vi "ATM_displayer.vi"(7 "Message":T1(ring), 9 "Amount":string, 10 "Users Info":string[](array[string])) -> (0 "Right Menu":cluster{string, string, string}, 1 "Left Menu":cluster{string, string, string}, 2 "Message display":string)   [LabVIEW 2025]
doc: "This VI handles the display of the ATM, the Left and Right Menu. It uses two inputs :\nMessage (required) : an Enum of 10 possible values\nUsers Info (optional) : a 1D Array of four strings constant"
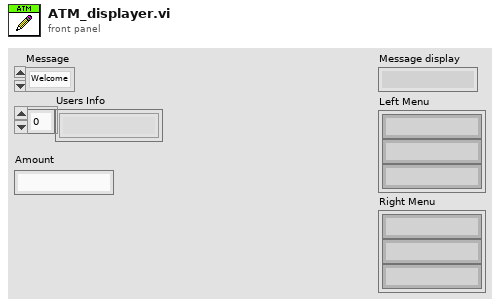
[diagram p1: front panel]
types:
  T1 = enum16{"Welcome", "Main Menu", "Account Verif Failed", "Session Terminate", "Deposit", "Deposit complete", "Withdrawal", "Withdrawal complete", "Withdrawal failed", "Balance Inquiry"}
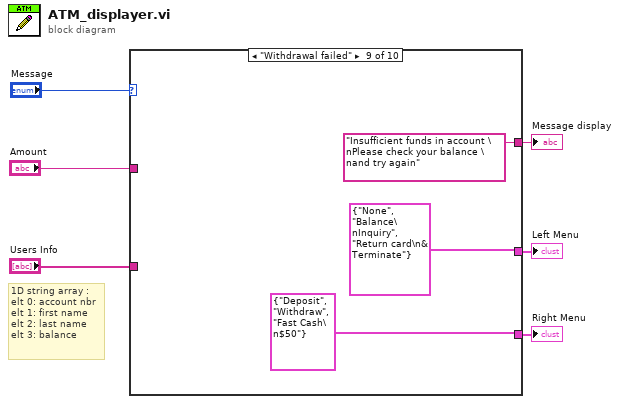
[diagram p0: block diagram]
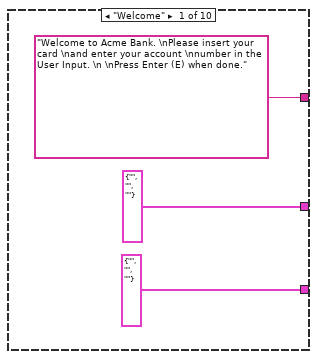
[diagram p2: hidden frame]
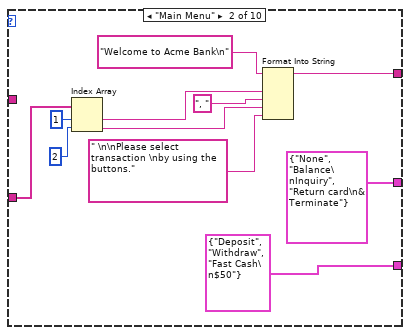
[diagram p3: hidden frame]
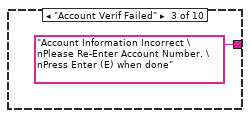
[diagram p4: hidden frame]
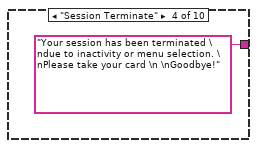
[diagram p5: hidden frame]
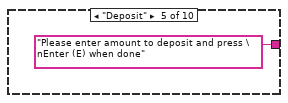
[diagram p6: hidden frame]
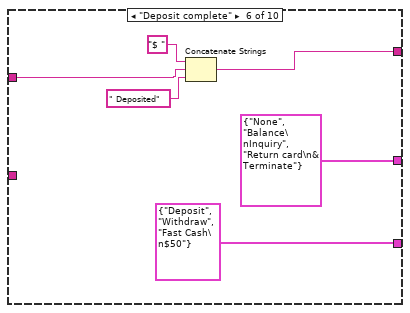
[diagram p7: hidden frame]
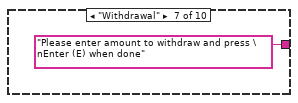
[diagram p8: hidden frame]
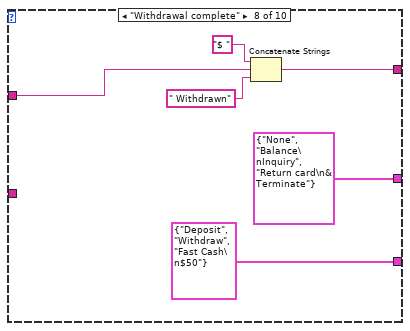
[diagram p9: hidden frame]
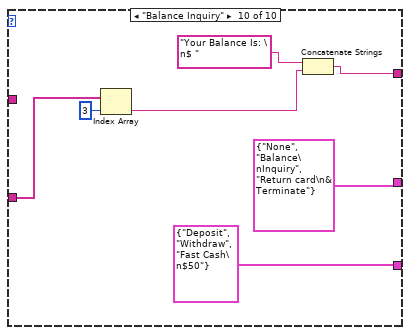
[diagram p10: hidden frame]
diagram:
  # "1D string array :\nelt 0: account nbr\nelt 1: first name\nelt 2: last name\nelt 3: balance"
  n1 = case shown="\"Withdrawal failed\"" "Message" {
    tunnel: ["Welcome to Acme Bank. \nPlease insert your card \nand enter your account \nnumber in the User Input. \n \nPress Enter (E) when done." w12 "Account Information Incorrect \nPlease Re-Enter Account Number. \nPress Enter (E) when done" "Your session has been terminated \ndue to inactivity or menu selection. \nPlease take your card \n \nGoodbye!" "Please enter amount to deposit and press \nEnter (E) when done" w26 "Please enter amount to withdraw and press \nEnter (E) when done" w32 "Insufficient funds in account \nPlease check your balance \nand try again" w42] -> w5
    tunnel: [cluster{string, string, string} {"", "", ""} cluster{string, string, string} {"None", "Balance\nInquiry", "Return card\n& Terminate"} _ _ _ cluster{string, string, string} {"None", "Balance\nInquiry", "Return card\n& Terminate"} _ cluster{string, string, string} {"None", "Balance\nInquiry", "Return card\n& Terminate"} cluster{string, string, string} {"None", "Balance\nInquiry", "Return card\n& Terminate"} cluster{string, string, string} {"None", "Balance\nInquiry", "Return card\n& Terminate"}] -> w4
    tunnel: [cluster{string, string, string} {"", "", ""} cluster{string, string, string} {"Deposit", "Withdraw", "Fast Cash\n$50"} _ _ _ cluster{string, string, string} {"Deposit", "Withdraw", "Fast Cash\n$50"} _ cluster{string, string, string} {"Deposit", "Withdraw", "Fast Cash\n$50"} cluster{string, string, string} {"Deposit", "Withdraw", "Fast Cash\n$50"} cluster{string, string, string} {"Deposit", "Withdraw", "Fast Cash\n$50"}] -> w3
    tunnel: "Users Info" -> [_ w20 _ _ _ _ _ _ _ w45]
    tunnel: "Amount" -> [_ _ _ _ _ w28 _ w31 _ _]
    frame "Welcome" {
    }
    frame "Main Menu" {
      n2 = Index Array(array=w20, index #1=1 ("index"), index #2=2 ("index")) -> (element #1=w16:string, element #2=w14:string)
      n3 = Format Into String(initial string="Welcome to Acme Bank\n", w16, ", " ("input 2"), w14, " \n\nPlease select transaction \nby using the buttons." ("input 4")) -> (resulting string=w12:string)  [unwired: 2 in, 1 out]
    }
    frame "Account Verif Failed" {
    }
    frame "Session Terminate" {
    }
    frame "Deposit" {
    }
    frame "Deposit complete" {
      n4 = Concatenate Strings("$ " ("string"), w28, " Deposited" ("string")) -> (w26:string)
    }
    frame "Withdrawal" {
    }
    frame "Withdrawal complete" {
      n5 = Concatenate Strings("$ " ("string"), w31, " Withdrawn" ("string")) -> (w32:string)
    }
    frame "Withdrawal failed" {
    }
    frame "Balance Inquiry" {
      n6 = Index Array(array=w45, index=3) -> (element=w44:string)
      n7 = Concatenate Strings("Your Balance Is: \n$ ", w44) -> (w42:string)
    }
  }
  "Message display" <- w5
  "Left Menu" <- w4
  "Right Menu" <- w3
